vi "Read MeasType.vi"(8 "error in (no error)":errorcluster, 11 "ChanGrp in":refnum<class "ChanGrp.lvclass">) -> (0 "error out":errorcluster, 2 "MeasType":T1, 3 "ChanGrp out":refnum<class "ChanGrp.lvclass">)   [LabVIEW 2012, in "Configuration Grandmaster.lvlib" / "ChanGrp.lvclass"]
uses:
  ChanGrp.lvclass
  Custom Ctrls/ge_MeasType.ctl
  ChanGrp.lvclass/ChanGrp.ctl
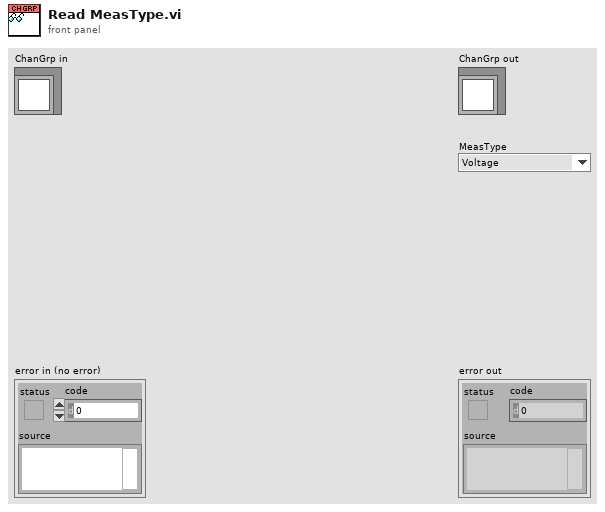
[diagram p1: front panel]
types:
  T1 = typedef "ge_MeasType.ctl" = enum16{"Voltage", "Frequency", "Tachometer", "Dynamic", "Thermocouple", "RTD", "Strain", "Current", "Resistance"}
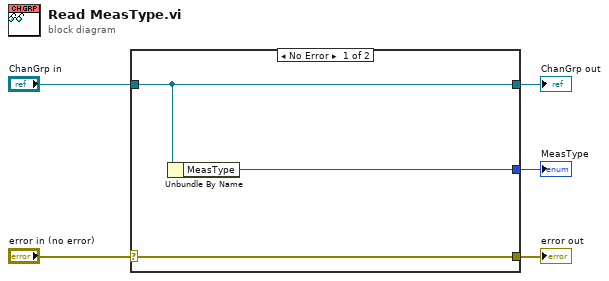
[diagram p0: block diagram]
diagram:
  n1 = case shown="No Error" "error in (no error)" {
    selector: "error in (no error)" -> [w8 w9]
    tunnel: [w8 w9] -> w4
    tunnel: [w7 w10] -> w2
    tunnel: "ChanGrp in" -> [w7 w10]
    tunnel: [w6 _] -> w1
    frame No Error {
      n2 = Unbundle By Name(w7) -> ("MeasType"=w6:T1)
    }
    frame Error {
    }
  }
  "error out" <- w4
  "ChanGrp out" <- w2
  "MeasType" <- w1
